vi "SignalGenerator_8.vi"(10 "Phase":fxp<+,64,64>[](array[numeric])=[0.0, 0.0, 0.0, 0.0, 0.0, 0.0, 0.0, 0.0], 11 "reset":bool) -> (1 "Sine out":fxp<+/-,16,0>[](array[numeric]), 2 "Cosine out":fxp<+/-,16,0>[](array[numeric]))   [LabVIEW 2013]
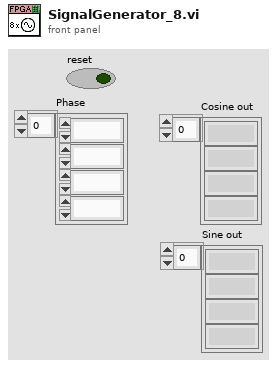
[diagram p1: front panel]
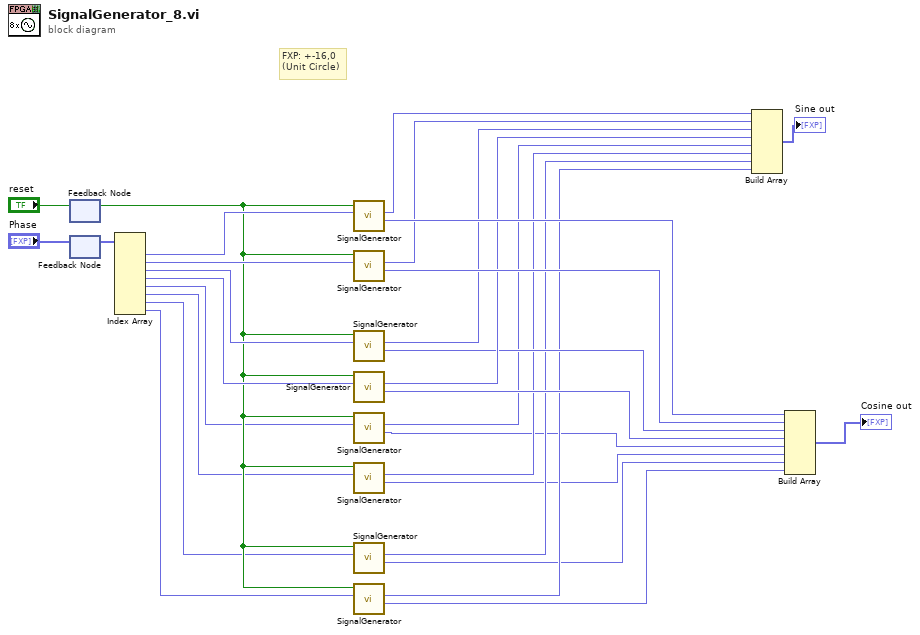
[diagram p0: block diagram]
diagram:
  # "FXP: +-16,0\n(Unit Circle)"
  n1 = feedback #1() -> (w13:bool)  [unwired: 1 in]
  n2 = feedback-in #1("reset") -> ()
  n3 = feedback #2() -> (w24:fxp<+,64,64>[])  [unwired: 1 in]
  n4 = feedback-in #2("Phase") -> ()
  n5 = Index Array(array=w24) -> (element #1=w22:fxp<+,64,64>, element #2=w28:fxp<+,64,64>, element #3=w27:fxp<+,64,64>, element #4=w26:fxp<+,64,64>, element #5=w12:fxp<+,64,64>, element #6=w11:fxp<+,64,64>, element #7=w10:fxp<+,64,64>, element #8=w9:fxp<+,64,64>)  [unwired: 8 in]
  n6 = call "SignalGenerator.vi"("phase"=w22, "Reset"=w13) -> ("Cos"=w20:fxp<+/-,16,0>, "Sin"=w21:fxp<+/-,16,0>)  [unwired: 7 in, 1 out]
  n7 = call "SignalGenerator.vi"("phase"=w28, "Reset"=w13) -> ("Cos"=w18:fxp<+/-,16,0>, "Sin"=w19:fxp<+/-,16,0>)  [unwired: 7 in, 1 out]
  n8 = call "SignalGenerator.vi"("phase"=w27, "Reset"=w13) -> ("Cos"=w15:fxp<+/-,16,0>, "Sin"=w17:fxp<+/-,16,0>)  [unwired: 7 in, 1 out]
  n9 = call "SignalGenerator.vi"("phase"=w26, "Reset"=w13) -> ("Cos"=w14:fxp<+/-,16,0>, "Sin"=w16:fxp<+/-,16,0>)  [unwired: 7 in, 1 out]
  n10 = call "SignalGenerator.vi"("phase"=w12, "Reset"=w13) -> ("Cos"=w4:fxp<+/-,16,0>, "Sin"=w8:fxp<+/-,16,0>)  [unwired: 7 in, 1 out]
  n11 = call "SignalGenerator.vi"("phase"=w11, "Reset"=w13) -> ("Cos"=w3:fxp<+/-,16,0>, "Sin"=w7:fxp<+/-,16,0>)  [unwired: 7 in, 1 out]
  n12 = call "SignalGenerator.vi"("phase"=w10, "Reset"=w13) -> ("Cos"=w2:fxp<+/-,16,0>, "Sin"=w6:fxp<+/-,16,0>)  [unwired: 7 in, 1 out]
  n13 = call "SignalGenerator.vi"("phase"=w9, "Reset"=w13) -> ("Cos"=w1:fxp<+/-,16,0>, "Sin"=w5:fxp<+/-,16,0>)  [unwired: 7 in, 1 out]
  n14 = Build Array(w21, w19, w17, w16, w8, w7, w6, w5) -> (→"Sine out":fxp<+/-,16,0>[])
  n15 = Build Array(w20, w18, w15, w14, w4, w3, w2, w1) -> (→"Cosine out":fxp<+/-,16,0>[])
